vi "HRTF-Read Responses.vi"(2 "State":T1, 7 "filestem":string, 11 "error in (no error)":errorcluster) -> (6 "time":cluster{"offset":dbl, "dx":dbl, "Y":dbl[][]}, 8 "crosscorr":cluster{"offset":dbl, "dx":dbl, "Y":dbl[][]}, 13 "phase":cluster{"offset":dbl, "dx":dbl, "Y":dbl[][]}, 14 "mag":cluster{"offset":dbl, "dx":dbl, "Y":dbl[][]}, 15 "error out":errorcluster)   [LabVIEW 2015]
uses:
  Typedefs/HRTF-State.ctl
  <vilib>/Analysis/2dsp.llb/Complex FFT.vi
  <vilib>/Analysis/2dsp.llb/Inverse Real FFT.vi
  Utility VIs/Math VIs/FFT x(t) to dB,Degrees (1D).vi
  Utility VIs/Conversion VIs/Create Waveform Cluster (2D).vi
  PXI DAQ VIs/Utility VIs/Array Dimensions (2D).vi
  <vilib>/Analysis/NI_AALPro.lvlib
panel:
  out "error out":errorcluster
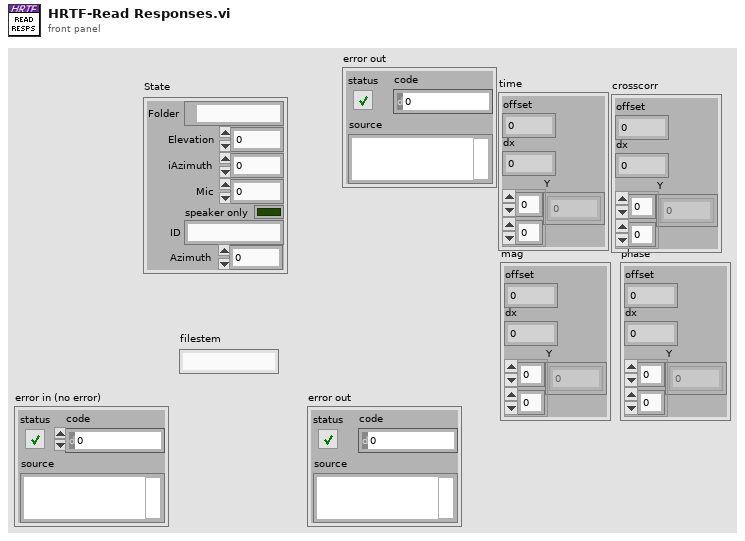
[diagram p1: front panel]
types:
  T1 = typedef "HRTF-State.ctl" = cluster{"Folder":path, "Elevation":dbl, "iAzimuth":i32, "Mic":i32, "speaker only":bool, "ID":string, "Azimuth":dbl}
  T2 = typedef "HRTF-Parameters.ctl" = cluster{"Fs (Hz)":dbl, "atten (dB)":dbl, "Waveform":T3, "Freq Res (Hz)":dbl, "Order":i32, "Averages":i32, "seed":i64, "Window":T4}
  T3 = typedef "HRTF-Waveform.ctl" = enum16{"Chirp", "MLS"}
  T4 = typedef "HRTF-Window.ctl" = cluster{"Type":T5, "Length (ms)":dbl, "Center (ms)":dbl}
  T5 = typedef "HRTF-Window Type.ctl" = enum16{"None", "Rectangle", "Hanning"}
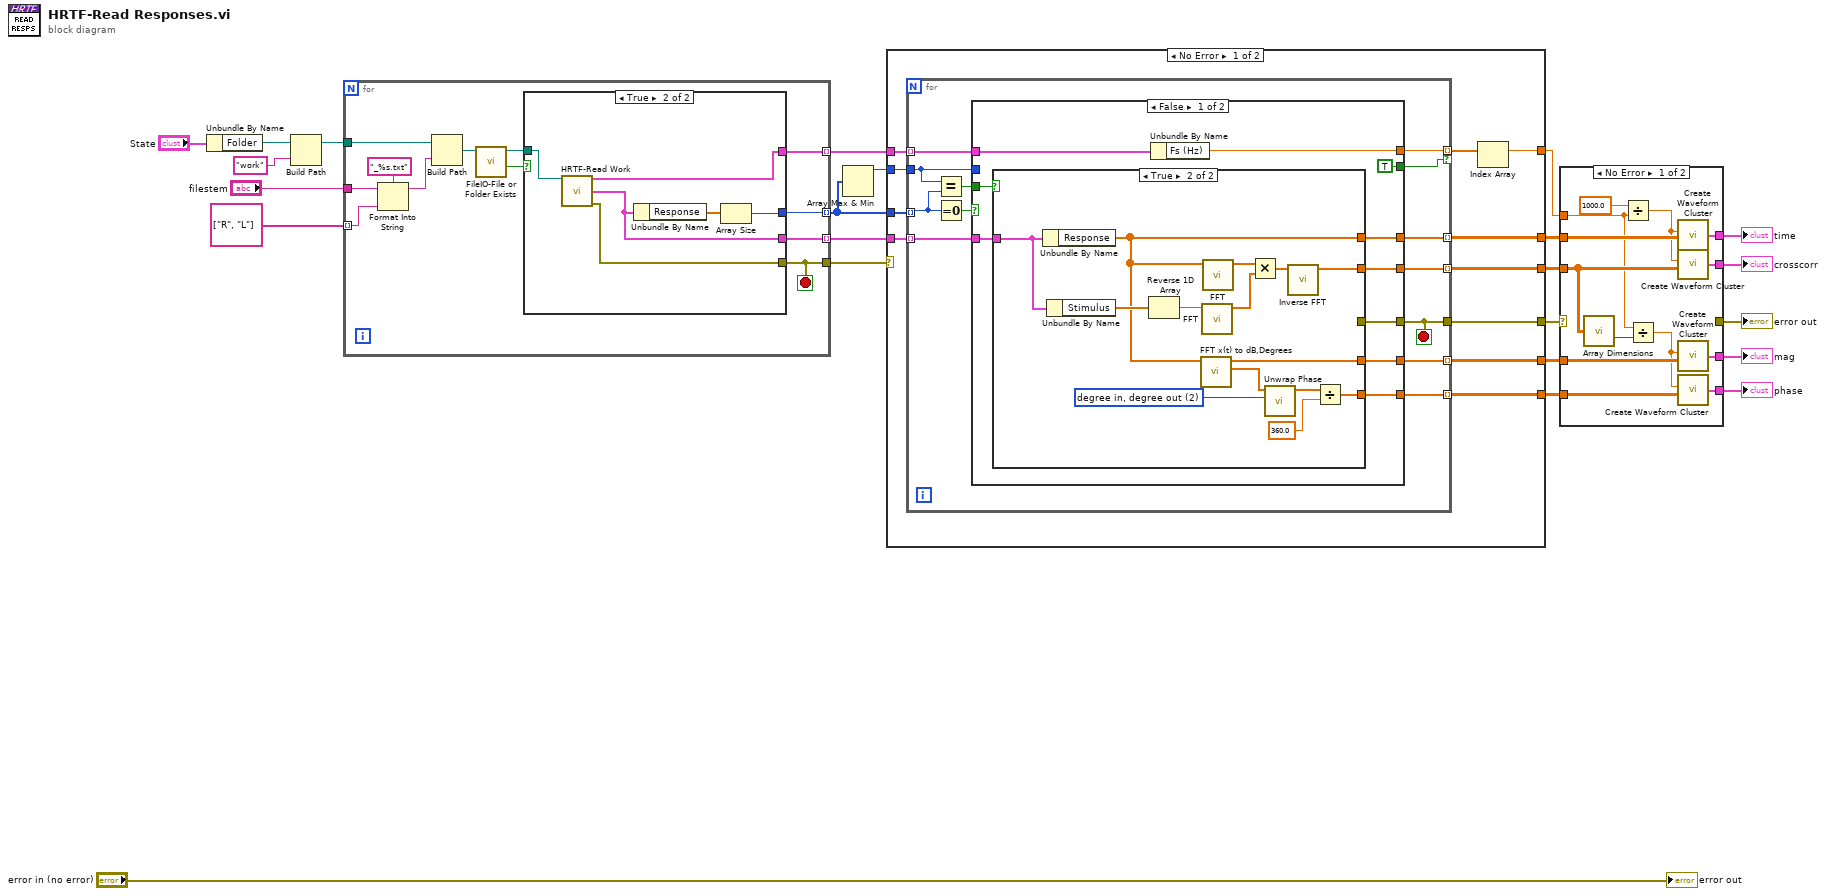
[diagram p0: block diagram]
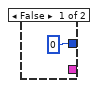
[diagram p2: hidden frame]
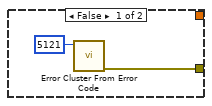
[diagram p4: hidden frame]
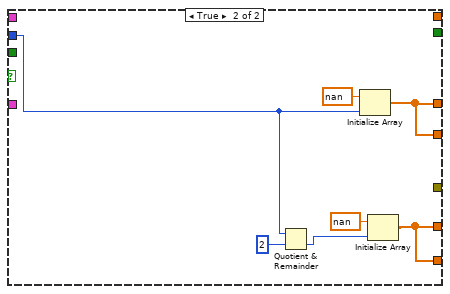
[diagram p5: hidden frame]
diagram:
  n1 = Unbundle By Name("State") -> ("Folder"=w20:path)
  n2 = Build Path(base path=w20, name or relative path="work") -> (appended path=w4:path)
  n3 = for {
    tunnel: string[] ["R", "L"] -> [w33] mode=indexing
    tunnel: w4 -> [w32]
    tunnel: "filestem" -> [w35]
    tunnel: [w30] -> w2 mode=indexing
    tunnel: [w29] -> w17 mode=indexing
    tunnel: [w24] -> w18
    tunnel: [w25] -> w15 mode=indexing
    stop <- w24 stop-if-true
    n4 = Format Into String(format string="_%s.txt", initial string=w35, w33) -> (resulting string=w31:string)  [unwired: 1 in, 1 out]
    n5 = Build Path(base path=w32, name or relative path=w31) -> (appended path=w28:path)
    n6 = call "FileIO-File or Folder Exists.vi"("path"=w28) -> ("Exists?"=w26:bool, "dup path"=w27:path)  [unwired: 7 in, 2 out]
    n7 = case shown="True" w26 {
      tunnel: [_ w40] -> w30
      tunnel: w27 -> [_ w42]
      tunnel: [_ w39] -> w29
      tunnel: [_ w41] -> w24
      tunnel: [0 w37] -> w25
      frame False {
      }
      frame True {
        n8 = call "HRTF-Read Work.vi"("path"=w42) -> ("Params"=w40:T2, "Result"=w39:cluster{"Stimulus":dbl[], "Response":dbl[]}, "error out"=w41:errorcluster)  [unwired: 12 in]
        n9 = Unbundle By Name(w39) -> ("Response"=w38:dbl[])
        n10 = Array Size(array=w38) -> (size(s)=w37:i32)
      }
    }
  }
  n11 = Array Max & Min(array=w15) -> (max value=w16:i32)  [unwired: 3 out]
  n12 = case shown="No Error" w18 {
    selector: w18 -> [_ w100]
    tunnel: w17 -> [w53 _]
    tunnel: w16 -> [w52 _]
    tunnel: w15 -> [w51 _]
    tunnel: [w50 w100] -> w14
    tunnel: [w49 _] -> w12
    tunnel: [w48 _] -> w13
    tunnel: [w47 _] -> w11
    tunnel: [w46 _] -> w10
    tunnel: w2 -> [w45 _]
    tunnel: [w43 _] -> w1
    frame No Error {
      n13 = for {
        tunnel: w53 -> [w62] mode=indexing
        tunnel: w52 -> [w65]
        tunnel: w51 -> [w64] mode=indexing
        tunnel: [w61] -> w49 mode=indexing
        tunnel: [w60] -> w48 mode=indexing
        tunnel: [w59] -> w47 mode=indexing
        tunnel: [w58] -> w46 mode=indexing
        tunnel: [w57] -> w50
        tunnel: w45 -> [w56] mode=indexing
        tunnel: [w55] -> w44 mode=indexing if=w54
        stop <- w57 stop-if-true
        n14 = Equal?(x=w65, y=w64) -> (x = y?=w63:bool)
        n15 = Equal To 0?(x=w64) -> (x = 0?=w66:bool)
        n16 = case shown="False" w66 {
          tunnel: w65 -> [_ w95]
          tunnel: w63 -> [w76 _]
          tunnel: w62 -> [w75 _]
          tunnel: [w74 w98] -> w61
          tunnel: [w73 w98] -> w60
          tunnel: [w72 w96] -> w59
          tunnel: [w71 w96] -> w58
          tunnel: [w70 _] -> w57
          tunnel: w56 -> [w69 _]
          tunnel: [w68 _] -> w55
          tunnel: [TRUE _] -> w54
          frame False {
            n17 = case shown="True" w76 {
              tunnel: w75 -> [_ w84]
              tunnel: [_ w82] -> w74
              tunnel: [_ w81] -> w73
              tunnel: [_ w80] -> w72
              tunnel: [_ w79] -> w71
              tunnel: [w77 _] -> w70
              frame False {
                n18 = call <vilib>:"Error Cluster From Error Code.vi"("error code (0)"=5121) -> ("error out"=w77:errorcluster)  [unwired: 8 in]
              }
              frame True {
                w90 = 2 items=["radian in, radian out", "radian in, degree out", "degree in, degree out", "degree in, radian out"] ("phase unit")
                n19 = Unbundle By Name(w84) -> ("Response"=w82:dbl[])
                n20 = Unbundle By Name(w84) -> ("Stimulus"=w87:dbl[])
                n21 = Reverse 1D Array(array=w87) -> (reversed array=w88:dbl[])
                n22 = call-poly "FFT x(t) to dB,Degrees.vi"("X"=w82) -> ("+Freq Phase of FFT (degrees)"=w91:dbl[], "+Freq. Mag of FFT (dB rms)"=w80:dbl[])  [unwired: 8 in, 1 out]
                n23 = call-poly <vilib>:"FFT.vi"("X"=w88) -> ("FFT {X}"=w89:cdb[])  [unwired: 9 in, 1 out]
                n24 = call-poly <vilib>:"FFT.vi"("X"=w82) -> ("FFT {X}"=w86:cdb[])  [unwired: 9 in, 1 out]
                n25 = Multiply(x=w86, y=w89) -> (x*y=w85:cdb[])
                n26 = call <vilib>:"Unwrap Phase.vi"("phase unit"=w90, "Phase"=w91) -> ("Unwrapped Phase"=w92:dbl[])  [unwired: 8 in, 1 out]
                n27 = call-poly <vilib>:"Inverse FFT.vi"("FFT {X}"=w85) -> ("X"=w81:dbl[])  [unwired: 9 in, 1 out]
                n28 = Divide(x=w92, y=360.0) -> (x/y=w79:dbl[])
              }
            }
            n29 = Unbundle By Name(w69) -> ("Fs (Hz)"=w68:dbl)
          }
          frame True {
            n30 = Quotient & Remainder(x=w95, y=2) -> (floor(x/y)=w93:i32)  [unwired: 1 out]
            n31 = Initialize Array(nan, w95) -> (w98:dbl[])
            n32 = Initialize Array(nan, w93) -> (w96:dbl[])
          }
        }
      }
      n33 = Index Array(array=w44) -> (element=w43:dbl)  [unwired: 1 in]
    }
    frame Error {
    }
  }
  n34 = case shown="No Error" w14 {
    selector: w14 -> [_ w114]
    tunnel: w13 -> [w104 _]
    tunnel: w12 -> [w113 _]
    tunnel: w11 -> [w112 _]
    tunnel: w10 -> [w111 _]
    tunnel: [w110 _] -> w9
    tunnel: [w109 _] -> w8
    tunnel: [w108 _] -> w7
    tunnel: [w107 _] -> w6
    tunnel: [_ w114] -> w5
    tunnel: w1 -> [w102 _]
    frame No Error {
      n35 = call-poly "Array Dimensions.vi"("2D Array"=w104) -> ("# columns"=w103:i32)  [unwired: 13 in, 1 out]
      n36 = Divide(x=1000.0, y=w102) -> (x/y=w105:dbl)
      n37 = Divide(x=w102, y=w103) -> (x/y=w101:dbl)
      n38 = call-poly "Create Waveform Cluster.vi"("dx"=w105, "Array"=w113) -> ("waveform cluster"=w110:cluster{"offset":dbl, "dx":dbl, "Y":dbl[][]})  [unwired: 3 in]
      n39 = call-poly "Create Waveform Cluster.vi"("dx"=w105, "Array"=w104) -> ("waveform cluster"=w109:cluster{"offset":dbl, "dx":dbl, "Y":dbl[][]})  [unwired: 3 in]
      n40 = call-poly "Create Waveform Cluster.vi"("dx"=w101, "Array"=w112) -> ("waveform cluster"=w108:cluster{"offset":dbl, "dx":dbl, "Y":dbl[][]})  [unwired: 3 in]
      n41 = call-poly "Create Waveform Cluster.vi"("dx"=w101, "Array"=w111) -> ("waveform cluster"=w107:cluster{"offset":dbl, "dx":dbl, "Y":dbl[][]})  [unwired: 3 in]
    }
    frame Error {
    }
  }
  "time" <- w9
  "mag" <- w7
  "phase" <- w6
  "crosscorr" <- w8
  "error out" <- w5
  "error out" <- "error in (no error)"
